vi "move to 2nd screen.vi"   [LabVIEW 2011]
doc: "Moves the selected IMAQ window to a second screen contected to the PC."
uses:
  <vilib>/express/express arith-compare/Formula/XNode/ExpressFormulaBlockNode.xnode
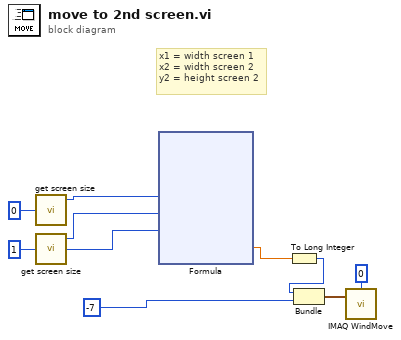
[diagram p0: block diagram]
diagram:
  # "x1 = width screen 1\nx2 = width screen 2\ny2 = height screen 2"
  n1 = call "get screen size.vi"("screen"=0) -> ("width"=w6:i16)  [unwired: 2 in, 2 out]
  n2 = call "get screen size.vi"("screen"=1) -> ("height"=w4:i16, "width"=w5:i16)  [unwired: 2 in, 1 out]
  n3 = xnode "Formula"("x1"=w6, "x2"=w5, "y2"=w4) -> ("Result"=w3:dbl)  [unwired: 1 in, 1 out]
  n4 = To Long Integer(number=w3) -> (32bit integer=w2:i32)
  n5 = Bundle(w2, "x"=-7) -> (w9:cluster{i32, "x":i32})  [unwired: 1 in]
  n6 = call "IMAQ WindMove"("Window Number (0...15)"=0, "Coordinates (screen)"=w9) -> ()  [unwired: 3 in, 2 out]
